vi "beginTableWith2ndStikerPlay.vi"(8 "error in (no error)":errorcluster, 10 "Game":refnum<class "Game.lvclass">, 11 "TableWith2ndStrikerPlay in":refnum<class "TableWith2ndStrikerPlay.lvclass">) -> (0 "error out":errorcluster, 2 "BeginTableWith2ndStriker?":bool, 3 "TableWith2ndStrikerPlay out":refnum<class "TableWith2ndStrikerPlay.lvclass">)   [LabVIEW 2021, in "TableWith2ndStrikerPlay.lvclass"]
uses:
  TableWith2ndStrikerPlay.lvclass
  Game_class/Game.lvclass
  Referee_class/command_interpreted.ctl
  Team_class/OffensivePlay.ctl
  Robot_class/roles.ctl
  Game_class/Game.lvclass/Game.ctl
  Referee_class/Referee.lvclass/Referee.ctl
  Object_class/Object.lvclass/Object.ctl
  Parameters_class/Parameters.lvclass/Parameters.ctl
  Team_class/Team.lvclass/Team.ctl
  Game_class/Read Referee.vi
  Game_class/Read Utilities.lvclass.vi
  Game_class/Read BallRef.vi
  Game_class/Read Parameters.lvclass.vi
  Game_class/Read FieldRef.vi
  Game_class/Read OffensiveTeam.vi
  Team_class/Read RobotRef.vi
  Parameters_class/Read AttakingOurselves.vi
  Object_class/Read x.vi
  Object_class/Read y.vi
  Referee_class/Read command_interpreted.vi
  Team_class/Read OffensivePlay.vi
  Ally_class/Ally.lvclass
  D:/RoboIme/horie/SSL_AI/Team_class/Team.lvclass
  Ball_class/Ball.lvclass
  D:/RoboIme/horie/SSL_AI/Object_class/Object.lvclass
  Robot_class/Robot.lvclass
  Referee_class/Referee.lvclass
  Utilities_class/Utilities.lvclass
  Parameters_class/Parameters.lvclass
  Field_class/Field.lvclass
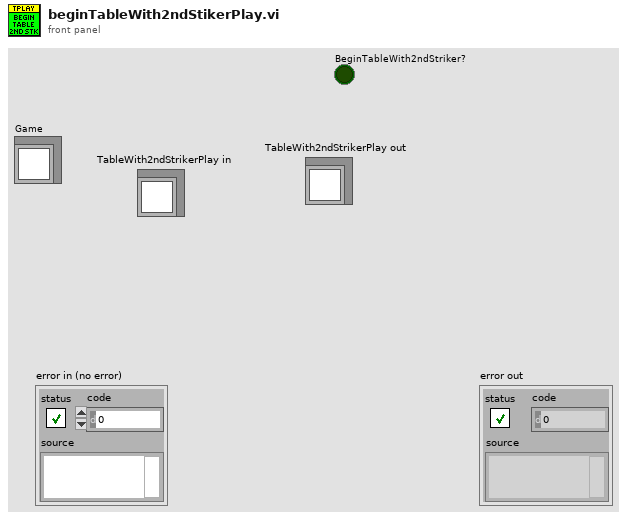
[diagram p1: front panel]
types:
  T1 = typedef "roles.ctl" = enum16{"SimpleBallPlacement", "BallPlacementAllyPasser", "BallPlacementAllyReceiver", "BallPlacementEnemy", "5Robots5th", "PassBestReceiver", "5Robots4th", "5Robots3rd", "5Robots2nd", "5Robots1st", "PassBestRobot", "WaitPass", "ABCThirdKicker", "ABCFirstKicker", "ABCSecondKicker", "Tabler", "TableFinalizer", "PrepareRollToPassRoller", "PrepareRollToPassReceiver", "SimplePassRoll", "SimplePassRollReceiver", "PenaltyDefense", "PreparePassReceiver 2", "PreparePassReceiver 1", "PassObserver", "Timeout", "Goto", "ZigZag", "None", "BallOutOfField", "DefenderArea", "Duelist", "AttackerStop", "FollowAttacker", "KeeperRole", "KickPenalty", "AttackerAimGoal", "AttackerBlock", "Marker", "Halt", "Shoot", "PassKicker", "PassReceiver", "TestRole", "PenaltyAttacker"}
  T2 = typedef "OffensivePlay.ctl" = enum16{"5RobotsPassGamePlay", "5PreparePassGame", "5RobotsKeeperGame", "KeeperPassToStriker", "5RobotsNormalGamePlay", "PrepareKeeperPass", "ACBPass", "ABCPass", "PrepareTriplePass", "TableWithStriker", "TableWith2ndStrikerPlay", "PrepareDoublePass", "PrepareRollToPass", "SimplePass", "PreparePass", "PassToStriker", "BallOutOfField", "PassTo2ndStriker", "StopOffensive", "Prepare Penalty Enemy", "EnemyPossessionAtEnemyField", "EnemyPossesionAtOurField", "TestPlay", "PreparePenaltyAlly", "KickPenaltyAlly", "PrepareKickoffAlly", "PrepareKickoffEnemy", "IndirectEnemy", "DirectEnemy", "PreparePassInGame1", "NormalGame", "DirectKick", "Pass", "Halt", "Timeout", "PassPlay", "PenaltyEnemy"}
  T3 = typedef "command_interpreted.ctl" = enum16{"Goal Ally", "Goal Enemy", "Ball Placement Enemy", "Ball Placement Ally", "Normal Half Time", "Extra Time  Break", "Extra Half Time", "None", "Post Game", "PKA Normal Start", "Prepare Kickoff Ally", "PKE Normal Start", "Prepare Kickoff Enemy", "Force Start", "Halt", "Timeout", "Prepare Penalty Ally", "Prepare Penalty Enemy", "PPA NormalStart", "PPE Normal Start", "Indirect Free Ally", "Direct Free Enemy", "Direct Free Ally", "Indirect Free Enemy", "Stop"}
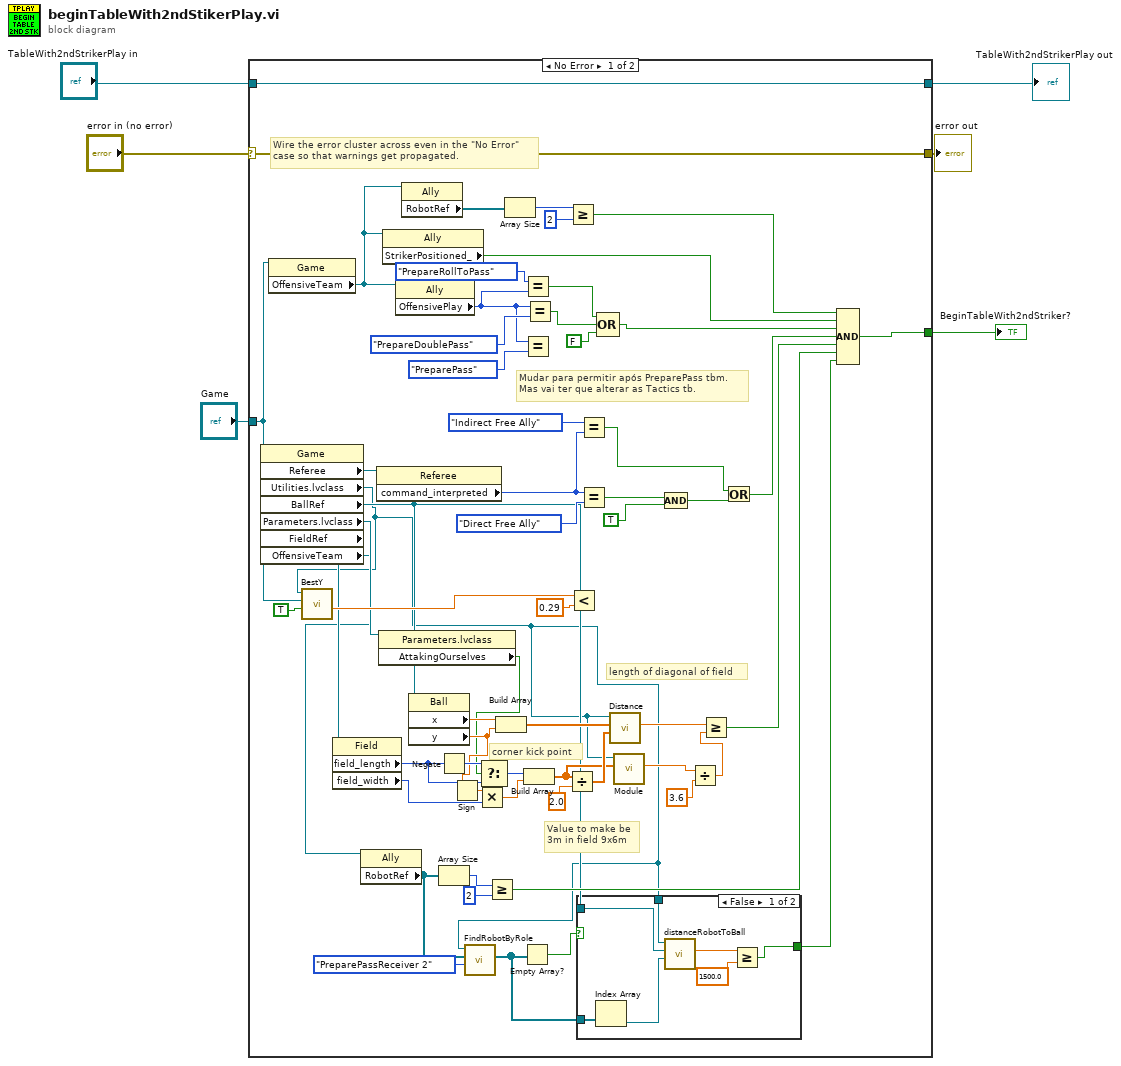
[diagram p0: block diagram]
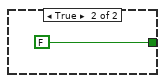
[diagram p2: hidden frame]
diagram:
  n1 = case shown="No Error" "error in (no error)" {
    selector: "error in (no error)" -> [w66 w77]
    tunnel: [w66 w77] -> w5
    tunnel: [w67 w76] -> w1
    tunnel: "TableWith2ndStrikerPlay in" -> [w67 w76]
    tunnel: "Game" -> [w58 _]
    tunnel: [w57 _] -> w3
    frame No Error {
      # "Mudar para permitir após PreparePass tbm.\nMas vai ter que alterar as Tactics tb."
      # "corner kick point"
      # "length of diagonal of field"
      # "Value to make be\n3m in field 9x6m"
      # "Wire the error cluster across even in the \"No Error\"\ncase so that warnings get propagated."
      n2 = property class="Game"(reference=w58) -> ("Referee"=w65:refnum<class "Referee.lvclass">, "Utilities.lvclass"=w9:refnum<class "Utilities.lvclass">, "BallRef"=w11:refnum<class "Ball.lvclass">, "Parameters.lvclass"=w25:refnum<class "Parameters.lvclass">, "FieldRef"=w23:refnum<class "Field.lvclass">, "OffensiveTeam"=w22:refnum<class "Ally.lvclass">)  [unwired: 1 in, 2 out]
      n3 = property class="Game"(reference=w58) -> ("OffensiveTeam"=w48:refnum<class "Ally.lvclass">)  [unwired: 1 in, 2 out]
      n4 = call "BestY.vi"("Utilities in"=w9, "Game"=w58, "inimigos"=TRUE) -> ("Gap kick"=w59:dbl)  [unwired: 2 in, 4 out]
      n5 = property class="Field"(reference=w23) -> ("field_length"=w38:i32, "field_width"=w37:i32)  [unwired: 1 in, 2 out]
      n6 = property class="Ally"(reference=w22) -> ("RobotRef"=w15:refnum<class "Robot.lvclass">[])  [unwired: 1 in, 2 out]
      n7 = property class="Referee"(reference=w65) -> ("command_interpreted"=w63:T3)  [unwired: 1 in, 2 out]
      n8 = property class="Parameters.lvclass"(reference=w25) -> ("AttakingOurselves"=w24:bool)  [unwired: 1 in, 2 out]
      n9 = property class="Ally"(reference=w48) -> ("StrikerPositioned_"=w56:bool)  [unwired: 1 in, 2 out]
      n10 = property class="Ally"(reference=w48) -> ("OffensivePlay"=w18:T2)  [unwired: 1 in, 2 out]
      n11 = property class="Ally"(reference=w48) -> ("RobotRef"=w47:refnum<class "Robot.lvclass">[])  [unwired: 1 in, 2 out]
      n12 = property class="Ball"(reference=w11) -> ("x"=w42:dbl, "y"=w36:dbl)  [unwired: 1 in, 2 out]
      n13 = Negate(x=w38) -> (-x=w40:i32)
      n14 = Array Size(array=w15) -> (size(s)=w21:i32)
      n15 = Sign(1:w36) -> (0:w35:dbl)
      n16 = call "FindRobotByRole.vi"("role"=roles."PreparePassReceiver 2", "RobotRef"=w15, "Utilities in"=w9) -> ("Robots"=w12:refnum<class "Robot.lvclass">[])  [unwired: 6 in, 2 out]
      n17 = Multiply(x=w35, y=w37) -> (x*y=w34:dbl)
      n18 = Select(t=w40, s=w24, f=w38) -> (s? t:f=w39:i32)
      n19 = Greater Or Equal?(x=w21, y=2) -> (x >= y?=w19:bool)
      n20 = Build Array(w42, w36) -> (w41:dbl[])
      n21 = Array Size(array=w47) -> (size(s)=w46:i32)
      n22 = Empty Array?(array=w12) -> (empty?=w13:bool)
      n23 = Equal?(x=OffensivePlay."PrepareRollToPass" ("OffensivePlay"), y=w18) -> (x = y?=w50:bool)
      n24 = Equal?(x=w18, y=OffensivePlay."PreparePass" ("OffensivePlay")) -> ()  [unwired: 1 out]
      n25 = Build Array(w39, w34) -> (w30:dbl[])
      n26 = Equal?(x=w18, y=OffensivePlay."PrepareDoublePass" ("OffensivePlay")) -> (x = y?=w51:bool)
      n27 = Divide(x=w30, y=2.0) -> (x/y=w31:dbl[])
      n28 = Greater Or Equal?(x=w46, y=2) -> (x >= y?=w44:bool)
      n29 = Less?(x=w59, y=0.29 ("Gap kick")) -> ()  [unwired: 1 out]
      n30 = case shown="False" w13 {
        tunnel: [w68 FALSE] -> w10
        tunnel: w12 -> [w74 _]
        tunnel: w9 -> [w72 _]
        tunnel: w11 -> [w71 _]
        frame False {
          n31 = Index Array(array=w74) -> (element=w73:refnum<class "Robot.lvclass">)  [unwired: 1 in]
          n32 = call "distanceRobotToBall.vi"("Robot"=w73, "Ball"=w71, "Utilities in"=w72) -> ("Distance Robot To Ball"=w70:dbl)  [unwired: 6 in, 2 out]
          n33 = Greater Or Equal?(x=w70, y=1500.0) -> (x >= y?=w68:bool)
        }
        frame True {
        }
      }
      n34 = Equal?(x=command_interpreted."Indirect Free Ally" ("command_interpreted"), y=w63) -> (x = y?=w54:bool)
      n35 = Equal?(x=w63, y=command_interpreted."Direct Free Ally" ("command_interpreted")) -> (x = y?=w55:bool)
      n36 = Compound Arithmetic op=OR(w50, w51, FALSE) -> (w49:bool)
      n37 = call "Distance.vi"("P1"=w31, "P2"=w41, "Utilities in"=w9) -> ("Distance"=w32:dbl)  [unwired: 6 in, 2 out]
      n38 = call "Module.vi"("2D vector"=w30, "Utilities in"=w9) -> ("Modulo"=w29:dbl)  [unwired: 7 in, 2 out]
      n39 = Compound Arithmetic op=AND(w55, TRUE ("value")) -> (w8:bool)
      n40 = Divide(x=w29, y=3.6) -> (x/y=w27:dbl)
      n41 = Greater Or Equal?(x=w32, y=w27) -> (x >= y?=w26:bool)
      n42 = Or(x=w54, y=w8) -> (x .or. y?=w43:bool)
      n43 = Compound Arithmetic op=AND(w44, w56, w49, w43, w26, w19, w10) -> (w57:bool)
    }
    frame Error {
    }
  }
  "error out" <- w5
  "BeginTableWith2ndStriker?" <- w3
  "TableWith2ndStrikerPlay out" <- w1
